vi "Hyperfactorial.vi"() -> ()   [LabVIEW 2022 SP3]
panel:
  out "Hyperfactorial":dbl format="%#_6f"
  in  "n":dbl
  # "Hyperfactorial:\nA hyperfactorial is defined as follows:\n         (1**1) x (2**2) x (3**3) x ... x (n**n)\nEnter a value for n to see the hyperfactorial\nof that integer. Note the value entered must \nbe a positive integer."
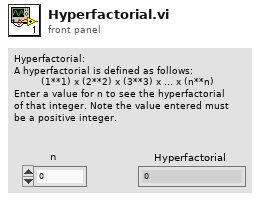
[diagram p1: front panel]
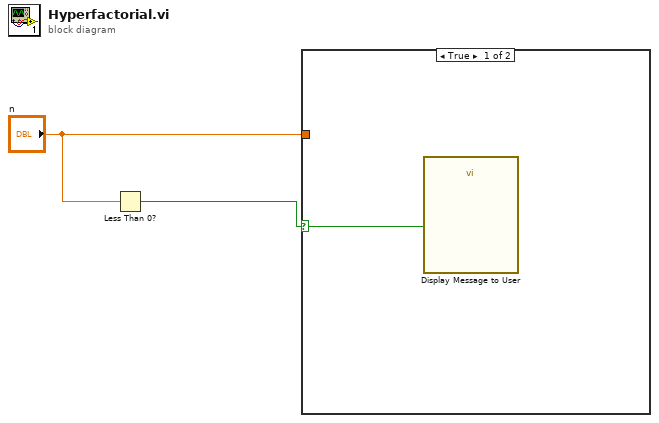
[diagram p0: block diagram]
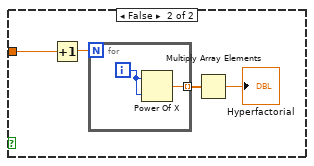
[diagram p2: hidden frame]
diagram:
  n1 = Less Than 0?(x="n") -> (x < 0?=w1:bool)
  n2 = case shown="True" w1 {
    selector: w1 -> [w3 _]
    tunnel: "n" -> [_ w4]
    frame True {
      n3 = call "Display Message to User"("Enable"=w3) -> ()  [unwired: 9 in, 2 out]
    }
    frame False {
      n4 = Increment(x=w4) -> (x+1=w5:dbl)
      n5 = for {
        N: w5 -> [_]
        tunnel: [w8] -> w6 mode=indexing
        i -> [w9]
        n6 = Power Of X(1:w9, 2:w9) -> (0:w8:dbl)
      }
      n7 = Multiply Array Elements(1:w6) -> (0:→"Hyperfactorial":dbl)
    }
  }
